vi "P4CMD Not A Source Control Reference.vi"(8 "error in (no error)":errorcluster, 10 "source control reference in":T1) -> (0 "error out":errorcluster, 2 "not a source control reference?":bool)   [LabVIEW 2017, in "NI_SCC_P4CMD.lvlib"]
doc: "Returns TRUE if <B>semaphore</B> is not a valid semaphore refnum."
uses:
  <vilib>/SourceControl/Providers/P4CMD/NI_SCC_P4CMD.lvlib
  <vilib>/SourceControl/sccapi/SCCAPI Refnum.ctl
  <vilib>/SourceControl/Providers/P4CMD/P4CMD Mgr Functions.ctl
  <vilib>/SourceControl/sccapi/NI_SCC.lvlib
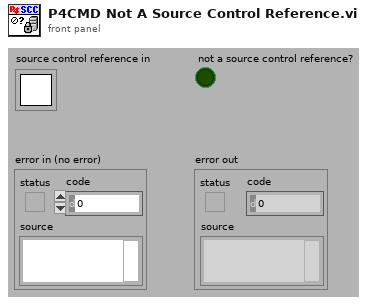
[diagram p1: front panel]
types:
  T1 = typedef "NI_SCC.lvlib/SCCAPI Refnum.ctl" = refnum<k1>
  T2 = typedef "NI_SCC_P4CMD.lvlib/P4CMD Mgr Functions.ctl" = enum16{"Init", "Open", "Set Config Opts", "Initialized?", "IsRefValid?", "Get Config Opts", "Get Global Commands", "Close", "Uninit"}
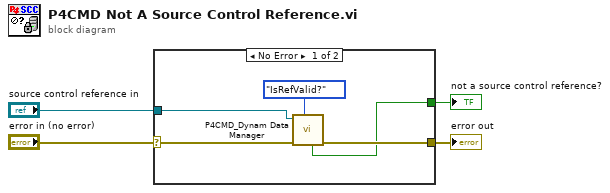
[diagram p0: block diagram]
diagram:
  n1 = case shown="No Error" "error in (no error)" {
    selector: "error in (no error)" -> [w9 w10]
    tunnel: [w8 w10] -> w4
    tunnel: [w5 _] -> w3
    tunnel: "source control reference in" -> [w7 _]
    frame No Error {
      n2 = call <vilib>:"P4CMD_Dynam Data Manager.vi"("function"=P4CMD_Mgr_Functions."IsRefValid?", "error in (no error)"=w9, "source control reference in"=w7) -> ("error out"=w8:errorcluster, "not a refnum?"=w5:bool)  [unwired: 3 in, 4 out]
    }
    frame Error {
      # "Return false if there was an error.  Since we never test refnum, we can't say if it's bad."
    }
  }
  "not a source control reference?" <- w3
  "error out" <- w4
